vi "hmp4000 Read Voltage Output.vi"(8 "error in (no error)":errorcluster, 11 "VISA resource name":refnum<visa-resource-name>) -> (0 "error out":errorcluster, 2 "Voltage Value":dbl format="%.3f", 3 "VISA resource name out":refnum<visa-resource-name>)   [LabVIEW 2022 SP3]
doc: "This VI queries the measured voltage value.\n\nAttribute:\nHMP4000_ATTR_MEASUREMENT_DC_VOLTAGE\n\nRemote-control command:\nMEASure[:VOLTage][:DC]?"
uses:
  Instance           1 35Saved   hmp4000 Read Voltage Output .vi
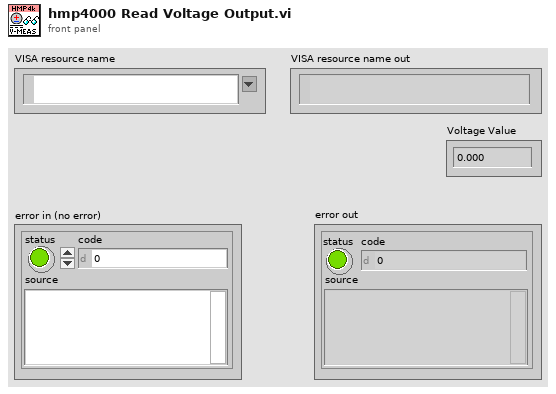
[diagram p1: front panel]
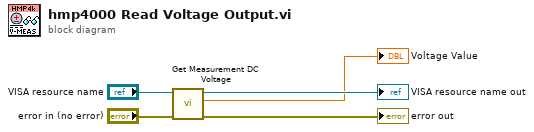
[diagram p0: block diagram]
diagram:
  n1 = call "Get Measurement DC Voltage"("error in (no error)"="error in (no error)", "instrument handle"="VISA resource name") -> ("error out"=→"error out":errorcluster, "Measurement DC Voltage"=→"Voltage Value":dbl, "instrument handle out"=→"VISA resource name out":refnum<visa-resource-name>)  [unwired: 7 in]
